vi "QGridLayout.vi"(8 "Error In":errorcluster, 11 "Post-Bundled Subclass":refnum<class "QGridLayout.lvclass">) -> (0 "Error Out":errorcluster, 3 "New QGridLayout":refnum<class "QGridLayout.lvclass">)   [LabVIEW 2014, in "QGridLayout.lvclass"]
doc: "LabVIEW-specific documentation is not yet available. See <b>http://doc.qt.io/qt-5/QGridLayout.html#QGridLayout</b>"
uses:
  QGridLayout.lvclass
  LQ Core/LQCoreEngine/_Internal/LQIdentity Registry Action.ctl
  LQ Core/LQIdentity/LQIdentity.lvclass/LQIdentity.ctl
  LQ Core/LQCoreEngine/LQCoreEngine.lvclass
  LQ Core/LQ Core.lvlib
  LQ Core/LQIdentity/LQIdentity.lvclass
panel:
  # "Copyright (c) 2016 Sze Howe Koh\n\nThis Source Code Form is subject to the terms of the Mozilla Public\nLicense, v. 2.0. If a copy of the MPL was not distributed with this\nfile, You can obtain one at http://mozilla.org/MPL/2.0/."
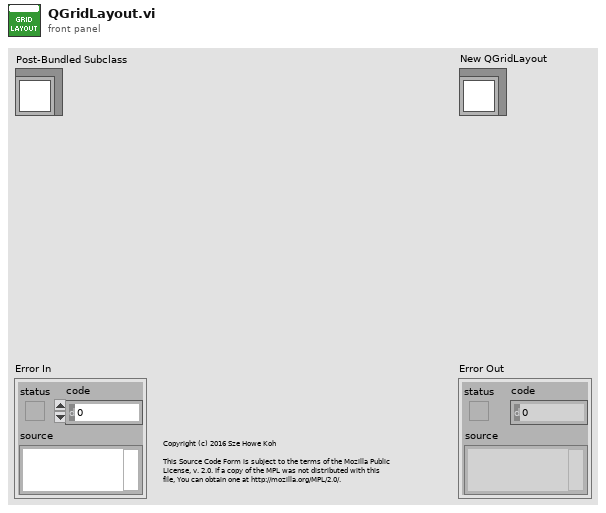
[diagram p1: front panel]
types:
  T1 = typedef "LQ Core.lvlib/LQCoreEngine.lvclass/LQIdentity Registry Action.ctl" = enum16{"Init", "Register LQIdentity", "Get LQIdentity Info", "Deregister LQIdentity"}
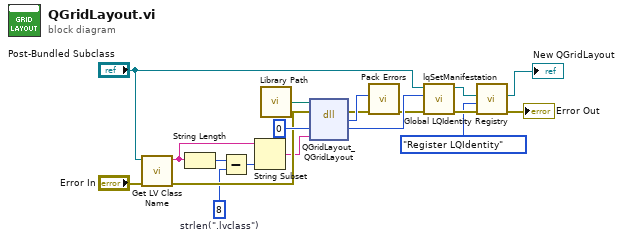
[diagram p0: block diagram]
diagram:
  w4 = 8  # strlen(".lvclass")
  n1 = call <vilib>:"Get LV Class Name.vi"("error in (no error)"="Error In", "object"="Post-Bundled Subclass") -> ("error out"=w6:errorcluster, "class name"=w2:string)  [unwired: 8 in]
  n2 = String Length(string=w2) -> (length=w5:i32)
  n3 = Subtract(x=w5, y=w4) -> (x-y=w3:i32)
  n4 = String Subset(string=w2, length (rest)=w3) -> (substring=w1:string)  [unwired: 1 in]
  n5 = call "Library Path.vi"() -> ("Library Path"=w17:path)
  n6 = dll-call lib="?" fn="QGridLayout_QGridLayout"(path in=w17, error in=w6, "_retVal"=u64 0 ("_instance"), "_className"=w1) -> (error out=w15:errorcluster, w16:i32, "_retVal"=w18:u64)  [unwired: 2 in, 1 out]
  n7 = call "Pack Errors.vi"("Error In"=w15, "Error Code"=w16) -> ("Error Out"=w14:errorcluster)  [unwired: 9 in]
  n8 = call "lqSetManifestation.vi"("Error In"=w14, "Manifestation"=w18, "LQIdentity in"="Post-Bundled Subclass") -> ("Error Out"=w12:errorcluster, "LQIdentity out"=w13:refnum<class "QGridLayout.lvclass">)  [unwired: 7 in]
  n9 = call "Global LQIdentity Registry.vi"("Error In"=w12, "Registry Action"=LQIdentity_Registry_Action."Register LQIdentity", "LQIdentity Info In"=w13) -> ("Error Out"=→"Error Out":errorcluster, "LQIdentity Info Out"=→"New QGridLayout":refnum<class "QGridLayout.lvclass">)  [unwired: 7 in]
